vi "test_definitions_module.vi"(7 "Delay time":dbl, 8 "error in (no error)":errorcluster, 9 "VISA resource in 19572":refnum<visa-resource-name>="COM6", 10 "VISA resource in 19052":refnum<visa-resource-name>="COM5", 11 "test mode":T1(ring)) -> (0 "error out":errorcluster, 3 "Mode parameters":T2 {"delay" format="%.2f"; "test time" format="%.2f"; "overlap" format="%.2f"; "2nd test" format="%.2f"; "1st test" format="%.2f"})   [LabVIEW 2015]
panel:
  # "in seconds"
  # "0 = HP--->GB \n1 = GB--->HP\n2 = HP only \n3 = GB only"
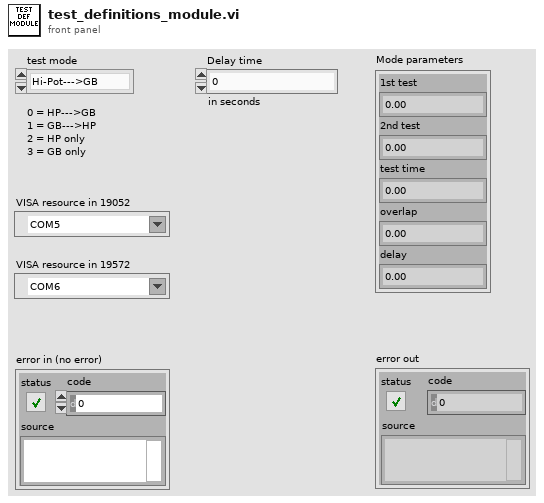
[diagram p1: front panel]
types:
  T1 = enum16{"Hi-Pot--->GB", "GB--->Hi-Pot", "Hi-Pot only", "GB only"}
  T2 = cluster{"1st test":dbl, "2nd test":dbl, "overlap":dbl, "test time":dbl, "delay":dbl}
  T3 = cluster{"T1 test":dbl, "T2 test":dbl, "overlap":dbl, "test time":dbl, "delay":dbl}
  T4 = cluster{"steps":u16[], "times":string[], "active steps":u16, "modes":string[], "Total time":dbl, "CONT.?":bool}
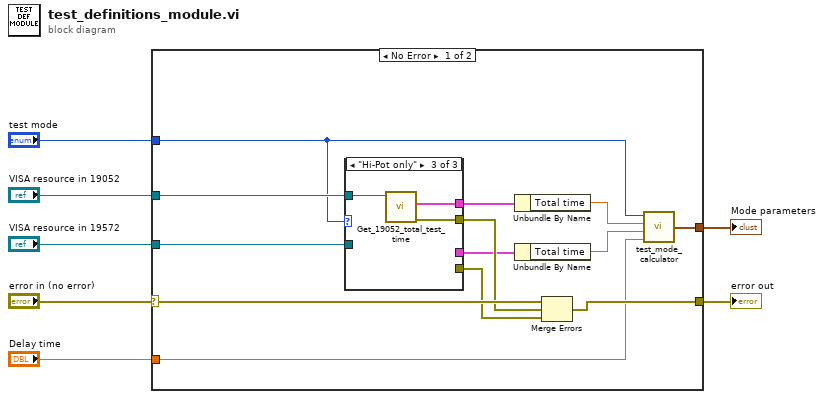
[diagram p0: block diagram]
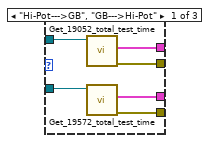
[diagram p2: hidden frame]
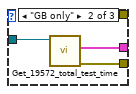
[diagram p3: hidden frame]
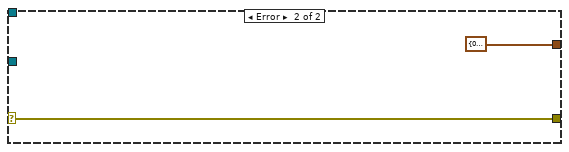
[diagram p4: hidden frame]
diagram:
  n1 = case shown="No Error" "error in (no error)" {
    selector: "error in (no error)" -> [w20 w34]
    tunnel: "VISA resource in 19052" -> [w19 _]
    tunnel: "VISA resource in 19572" -> [w18 _]
    tunnel: [w17 w34] -> w5
    tunnel: "Delay time" -> [w10 _]
    tunnel: "test mode" -> [w9 _]
    tunnel: [w8 T3 {"T1 test"=0.0, "T2 test"=0.0, "overlap"=0.0, "test time"=0.0, "delay"=0.0} ("Mode parameters")] -> w1
    frame No Error {
      n2 = case shown="\"Hi-Pot only\"" w9 {
        tunnel: w19 -> [w26 _ w32]
        tunnel: w18 -> [w25 w29 _]
        tunnel: [w24 w28 _] -> w16
        tunnel: [w23 _ w31] -> w15
        tunnel: [w22 w27 _] -> w12
        tunnel: [w21 _ w30] -> w11
        frame "Hi-Pot--->GB", "GB--->Hi-Pot" {
          n3 = call "Get_19052_total_test_time.vi"("VISA resource in"=w26) -> ("error out"=w23:errorcluster, "Data"=w21:T4)  [unwired: 8 in, 1 out]
          n4 = call "Get_19572_total_test_time.vi"("VISA resource in"=w25) -> ("error out"=w24:errorcluster, "Data"=w22:T4)  [unwired: 8 in, 1 out]
        }
        frame "GB only" {
          n5 = call "Get_19572_total_test_time.vi"("VISA resource in"=w29) -> ("error out"=w28:errorcluster, "Data"=w27:T4)  [unwired: 8 in, 1 out]
        }
        frame "Hi-Pot only" {
          n6 = call "Get_19052_total_test_time.vi"("VISA resource in"=w32) -> ("error out"=w31:errorcluster, "Data"=w30:T4)  [unwired: 8 in, 1 out]
        }
      }
      n7 = Unbundle By Name(w11) -> ("Total time"=w14:dbl)
      n8 = Unbundle By Name(w12) -> ("Total time"=w13:dbl)
      n9 = Merge Errors(w20, w15, w16) -> (w17:errorcluster)
      n10 = call "test_mode_calculator.vi"("Mode"=w9, "Hi-Pot test time"=w14, "GB test time"=w13, "Delay"=w10) -> ("Mode parameters"=w8:T3)  [unwired: 3 in]
    }
    frame Error {
    }
  }
  "error out" <- w5
  "Mode parameters" <- w1
